vi "0_SetupCameraAttributes (SubVI).vi"(8 "error in (no error)":errorcluster, 10 "Gain":dbl(slide)=4.875739644970414 scale=0.0..20.0, 11 "Camera session in":T1) -> (0 "error out":errorcluster, 3 "Camera session out":T1)   [LabVIEW 2016]
uses:
  <vilib>/userdefined/High Color/IMAQdx.ctl
  <vilib>/vision/driver/IMAQdx.llb/IMAQdx Attribute Visibility.ctl
  <vilib>/vision/driver/NI_Vision_Acquisition_Software.lvlib
  <resource>/objmgr/imaqdx.rc
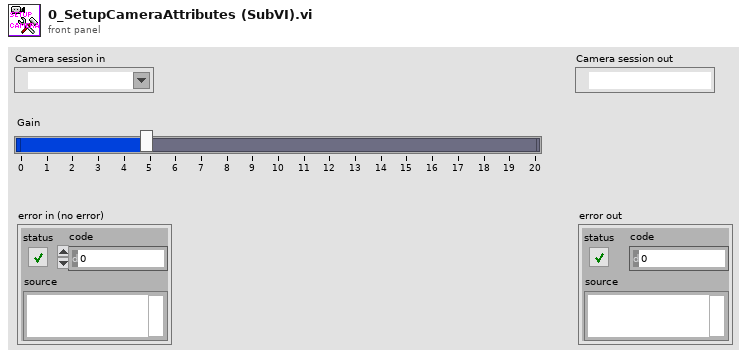
[diagram p1: front panel]
types:
  T1 = typedef "IMAQdx.ctl" = refnum<k21>
  T2 = typedef "NI_Vision_Acquisition_Software.lvlib/IMAQdx Attribute Visibility.ctl" = enum32{"Simple", "Intermediate", "Advanced"}
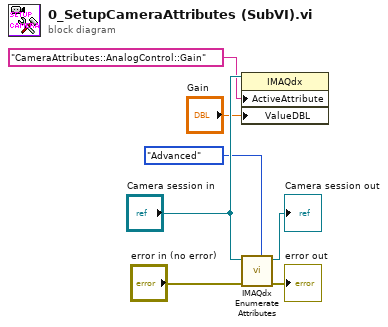
[diagram p0: block diagram]
diagram:
  n1 = property class="IMAQdx"(reference="Camera session in", "ActiveAttribute"="CameraAttributes::AnalogControl::Gain", "ValueDBL"="Gain") -> ()  [unwired: 1 in, 2 out]
  n2 = call <vilib>:"IMAQdx Enumerate Attributes.vi"("Visibility"=IMAQdx_Attribute_Visibility."Advanced", "error in"="error in (no error)", "Session In"="Camera session in") -> ("error out"=→"error out":errorcluster, "Session Out"=→"Camera session out":T1)  [unwired: 6 in, 1 out]
